vi "example1.vi"() -> ()   [LabVIEW 2015]
panel:
  in  "y":dbl
  out "Tank":dbl(slide) scale=-5.0..50.0
  in  "Slide":dbl(slide) scale=0.0..10.0
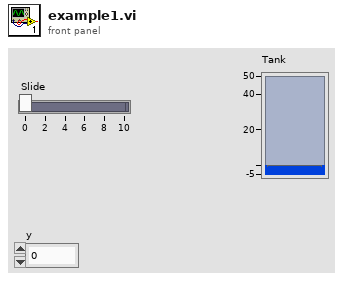
[diagram p1: front panel]
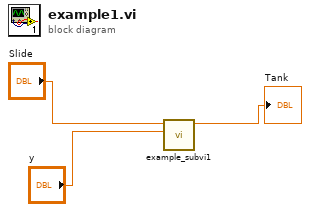
[diagram p0: block diagram]
diagram:
  n1 = call "example_subvi1.vi"("y"="y", "Slide"="Slide") -> ("Numeric"=→"Tank":dbl)  [unwired: 9 in]
